vi "BrowerFactory.vi"(8 "error in (no error)":errorcluster, 10 "BrowerIndex(0)":i32, 11 "ProjectBuilder in":refnum<class "ProjectBuilder.lvclass">) -> (0 "error out":errorcluster, 2 "BrowerComponent":refnum<class "BrowerComponent.lvclass">, 3 "ProjectBuilder out":refnum<class "ProjectBuilder.lvclass">)   [LabVIEW 2015, in "ProjectBuilder.lvclass"]
uses:
  ProjectBuilder.lvclass
  BrowerComponent/BrowerComponent/BrowerComponent.lvclass
  BrowerComponent/BrowerComposite/BrowerComposite.lvclass
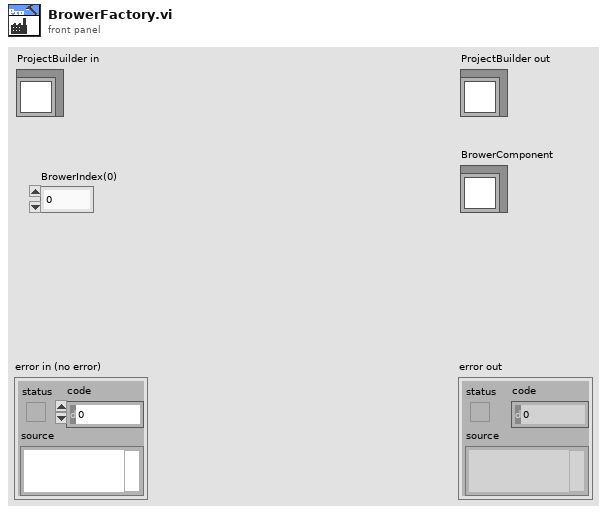
[diagram p1: front panel]
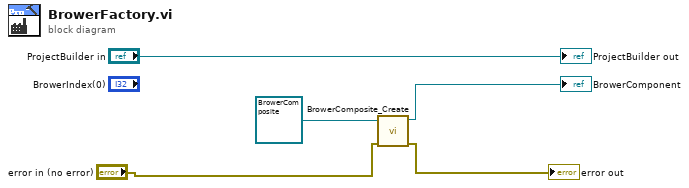
[diagram p0: block diagram]
diagram:
  n1 = call "BrowerComposite_Create.vi"("error in (no error)"="error in (no error)", "reference in"=refnum<class "BrowerComposite.lvclass"> refnum ("BrowerComposite")) -> ("error out"=→"error out":errorcluster, "reference out"=→"BrowerComponent":refnum<class "BrowerComposite.lvclass">)  [unwired: 8 in]
  "ProjectBuilder out" <- "ProjectBuilder in"
